vi "Test Loader.vi"() -> ()   [LabVIEW 2020]
uses:
  Models/Data Loader/Data Loader/Data Loader/Data Loader.lvclass
  C:/Program Files (x86)/National Instruments/LabVIEW 2020/vi.lib/ActorFramework/Actor/Actor.lvclass
  Models/Data Types/TDMS/TDMS.lvclass
  Models/Data Loader/Data Loader/Data Loader/Data Loader.lvclass/Data Loader.ctl
  Models/Data Loader/Data Load Interface/Data Load Interface Messages/Select File Msg/Select File Msg.lvclass/Select File Msg.ctl
  <vilib>/ActorFramework/Message Enqueuer/Message Enqueuer.lvclass/Message Enqueuer.ctl
  Models/Data Loader/Data Load Interface/Data Load Interface Messages/File Range Msg/File Range Msg.lvclass/File Range Msg.ctl
  Models/Data Loader/Data Load Interface/Data Load Interface Messages/Select Channel Msg/Select Channel Msg.lvclass/Select Channel Msg.ctl
  Models/Data Loader/Data Loader/Data Loader/Accessor/Write Data File.lvclass.vi
  <vilib>/ActorFramework/Message Enqueuer/Enqueue.vi
  Models/Data Loader/Data Load Interface/Data Load Interface Messages/Select File Msg/Select File Msg.lvclass
  C:/Program Files (x86)/National Instruments/LabVIEW 2020/vi.lib/ActorFramework/Message/Message.lvclass
  Models/Data Loader/Data Load Interface/Data Load Interface Messages/File Range Msg/File Range Msg.lvclass
  <vilib>/ActorFramework/Stop Msg/Stop Msg.lvclass
  Models/Data Loader/Data Load Interface/Data Load Interface Messages/Select Channel Msg/Select Channel Msg.lvclass
  <vilib>/ActorFramework/Message Priority Queue/Priority Enqueue.vi
  <vilib>/ActorFramework/Actor/Actor.lvclass
panel:
  in  "Combo Box":string(combo)
  in  "Stop":bool
  in  "end":dbl
  in  "index":dbl
  in  "File Path":path
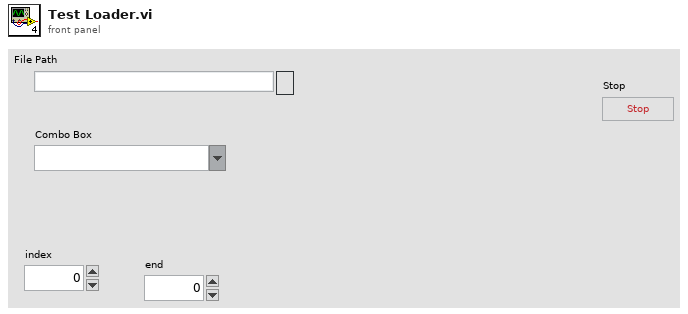
[diagram p1: front panel]
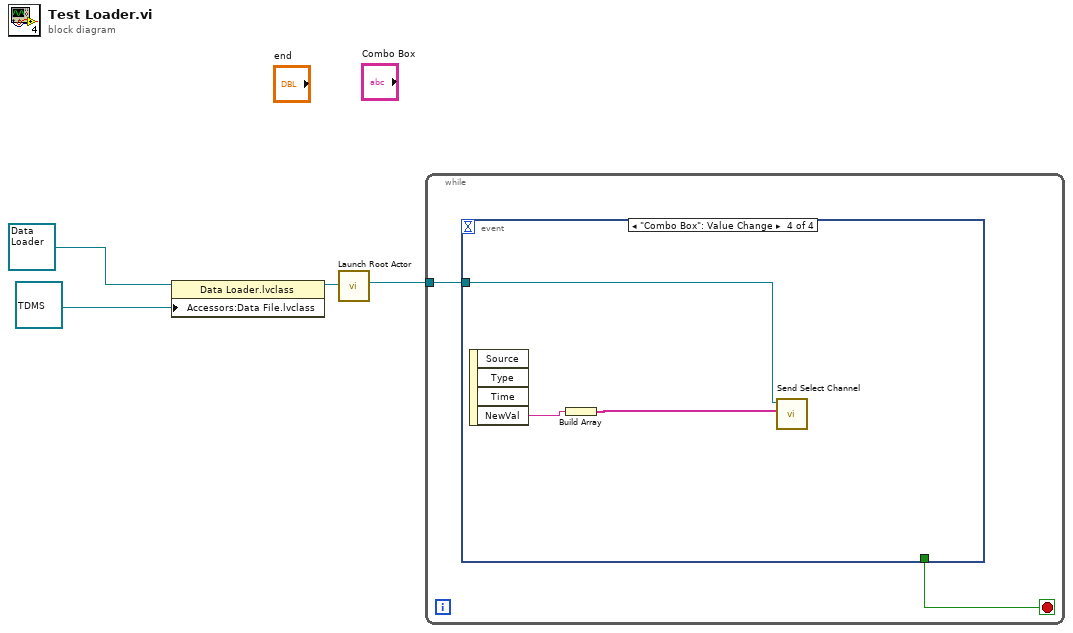
[diagram p0: block diagram]
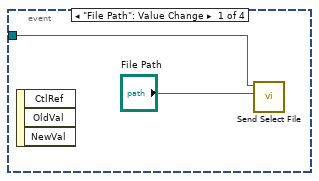
[diagram p2: hidden frame]
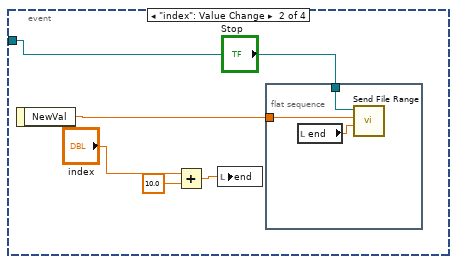
[diagram p3: hidden frame]
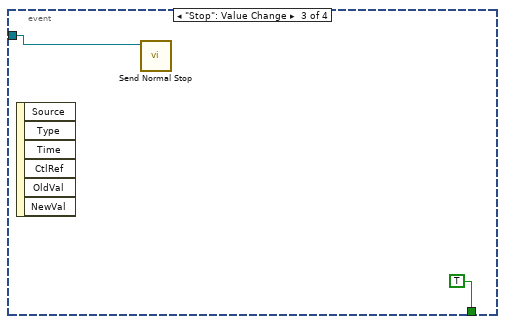
[diagram p4: hidden frame]
diagram:
  n1 = property class="Data Loader.lvclass"(reference=refnum<class "Data Loader.lvclass"> refnum ("Data Loader.lvlib:Data Loader.lvclass"), "Accessors:Data File.lvclass"=refnum<class "TDMS.lvclass"> refnum ("TDMS.lvclass")) -> (reference out=w2:refnum<class "Data Loader.lvclass">)  [unwired: 1 in, 1 out]
  n2 = call <vilib>:"Launch Root Actor.vi"("Actor"=w2) -> ("Actor's Enqueuer"=w4:refnum<class "Message Enqueuer.lvclass">)  [unwired: 9 in, 1 out]
  n3 = while {
    tunnel: w4 -> [w6]
    stop <- w5 stop-if-true
    n4 = event shown="[3] \"Combo Box\": Value Change" {
      selector: _ -> [_ _ _ _]
      dyn-events: _ -> [_ _ _ _]
      timeout: _ -> [_ _ _ _]
      tunnel: w6 -> [w8 w11 w18 w21]
      tunnel: [_ _ TRUE _] -> w5
      event "File Path": Value Change {
        n5 = event-data() -> ()  [unwired: 1 in, 3 out]
        n6 = call "Send Select File.vi"("File Path"="File Path", "Message Enqueuer"=w8) -> ()  [unwired: 8 in, 2 out]
      }
      event "index": Value Change {
        n7 = event-data() -> ("NewVal"=w10:dbl)  [unwired: 1 in]
        n8 = Add(x="index", y=10.0) -> (x+y=w12:dbl)
        n9 = local write "end"(w12) -> ()
        n10 = flat-sequence {
          tunnel: w11 -> [w16]
          tunnel: w10 -> [w15]
          frame #0 {
            n11 = local read "end"() -> (w14:dbl)
            n12 = call "Send File Range.vi"("End(%)"=w14, "start(%)"=w15, "Message Enqueuer"=w16) -> ()  [unwired: 7 in, 2 out]
          }
        }
      }
      event "Stop": Value Change {
        n13 = event-data() -> ()  [unwired: 1 in, 6 out]
        n14 = call <vilib>:"Send Normal Stop.vi"("Message Enqueuer"=w18) -> ()  [unwired: 10 in, 1 out]
      }
      event "Combo Box": Value Change {
        n15 = event-data() -> ("NewVal"=w20:string)  [unwired: 1 in, 3 out]
        n16 = Build Array(w20) -> (w19:string[])
        n17 = call "Send Select Channel.vi"("Select Channels"=w19, "Message Enqueuer"=w21) -> ()  [unwired: 8 in, 2 out]
      }
    }
  }
